vi "Set Buffer.vi"(6 "Set? [T]":bool=TRUE, 8 "error in (no error)":errorcluster, 11 "Carya Config":refnum<class "Carya Config (By Reference).lvclass">) -> (0 "error out":errorcluster, 3 "Carya Config out":refnum<class "Carya Config (By Reference).lvclass">)   [LabVIEW 2013, in "Carya Config (By Reference).lvclass"]
doc: "Copyright 2018, Carya Automatisering, Wiebe Walstra."
uses:
  Carya Config (By Reference).lvclass
  Carya Config (By Reference).lvclass/Carya Config (By Reference).ctl
  CConfig Buffer Type/CConfig Buffer Type.lvclass
  Carya Config.lvclass
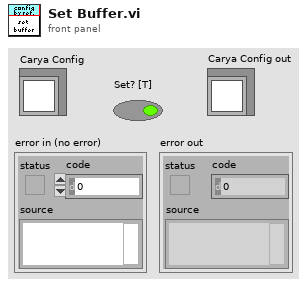
[diagram p1: front panel]
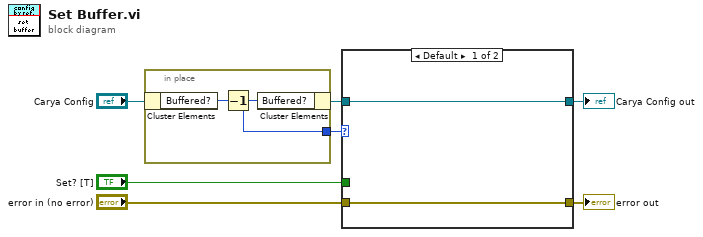
[diagram p0: block diagram]
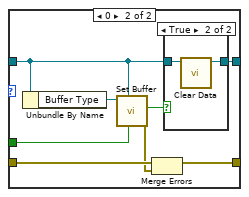
[diagram p2: hidden frame]
diagram:
  n1 = in-place {
    in-place-border: [w8] -> w2
    n2 = in-place-cluster #1("Carya Config") -> ("Buffered?"=w9:i32)
    n3 = Decrement(x=w9) -> (x-1=w8:i32)
    n4 = in-place-cluster #1("Buffered?"=w8) -> (w3:refnum<class "Carya Config (By Reference).lvclass">)
  }
  n5 = case shown="Default" w2 {
    tunnel: [w11 w19] -> w7
    tunnel: "error in (no error)" -> [w10 w18]
    tunnel: [w10 w17] -> w5
    tunnel: w3 -> [w11 w13]
    tunnel: "Set? [T]" -> [_ w12]
    frame Default {
    }
    frame 0 {
      n6 = Unbundle By Name(w13) -> ("Buffer Type"=w14:refnum<class "CConfig Buffer Type.lvclass">)
      n7 = call-dynamic "Set Buffer.vi"("Set? [T]"=w12, "Config in"=w13, "Carya Config (Buffer) in"=w14) -> ("error out"=w15:errorcluster, "Replace?"=w16:bool)  [unwired: 6 in, 1 out]
      n8 = Merge Errors(w18, w15) -> (w17:errorcluster)
      n9 = case shown="True" w16 {
        tunnel: [w20 w22] -> w19
        tunnel: w13 -> [w20 w21]
        frame False {
        }
        frame True {
          n10 = call "Clear Data.vi"("Carya Config in"=w21) -> ("Carya Config out"=w22:refnum<class "Carya Config (By Reference).lvclass">)  [unwired: 9 in, 1 out]
        }
      }
    }
  }
  "error out" <- w5
  "Carya Config out" <- w7
